vi "save_mpi_tdms.vi"(3 "System Information cluster":T1, 5 "Subject metadata cluster":T2, 7 "Device Name":tag="DAQ2", 8 "TxRxParams":T3={"sample rate"=1000000.0, "Transmit frequency"=25000.0, "Transmit amplitude"=1.577, "sample rate digital out"=40000.0, "TX cycles"=600, "sample rate DAQ1"=1000000.0, "Receive frequency"=75000.0, "Receive range"=1.0, "TX harmonics"=[50000.0, 75000.0, 100000.0, 125000.0, 150000.0, 175000.0, 200000.0, 225000.0]} {"TX harmonics" format="%#_6p"; "Receive frequency" format="%#_6p"; "sample rate DAQ1" format="%#_6p"; "sample rate digital out" format="%#_6p"; "Transmit frequency" format="%#_6p"; "sample rate" format="%#_6p"}, 9 "image dataset":string, 10 "Path":path, 11 "Cluster in":T4={"Magnitude meas."=[], "Phase meas."=[], "Shift meas."=[], "cw"=TRUE, "projections per image"=0, "ramp-up readouts"=0, "current sense type"="", "Number of pulses per image"=0, "Rotation enabled"=TRUE, "Rotary position"=[], "Baseline magnitude"=0.0, "Baseline phase"=0.0, "Wait readouts"=0, "Shift waveform type"="", "Shift enabled"=TRUE, "Time domain data"=[], "Motor pulse duration"=0.0, "Shift Amp pk"=0.0, "Shift DC offset"=0.0, "Notes"="", "Reconstructed image"=bytes[0], "Rotary encoder type"="", "Image start"=timestamp(0 s since 1904-01-01), "Image stop"=timestamp(0 s since 1904-01-01), "readouts per projection"=0, "Recon enabled"=FALSE, "Bidirectional shift"=FALSE, "Imager mode"="", "Shift delay"=0.0, "Shift frequency"=0.0, "Image time (calc)"=0.0, "Initial encoder position"=0.0, "Recon data"=[], "Trigger line values"=[], "Bed position"=0.0, "Sample image"=bytes[0], "Patch amplitude"=0.0, "Patch frequency"=0.0, "Patch phase"=0.0, "proj mag f2-f9"=[], "proj phase f2-f9"=[], "Tx waveform"=[], "Tx FFT mag"=[], "Tx FFT phase"=[], "Temps"=[]}) -> ()   [LabVIEW 2021]
uses:
  <resource>/objmgr/daqmx.rc
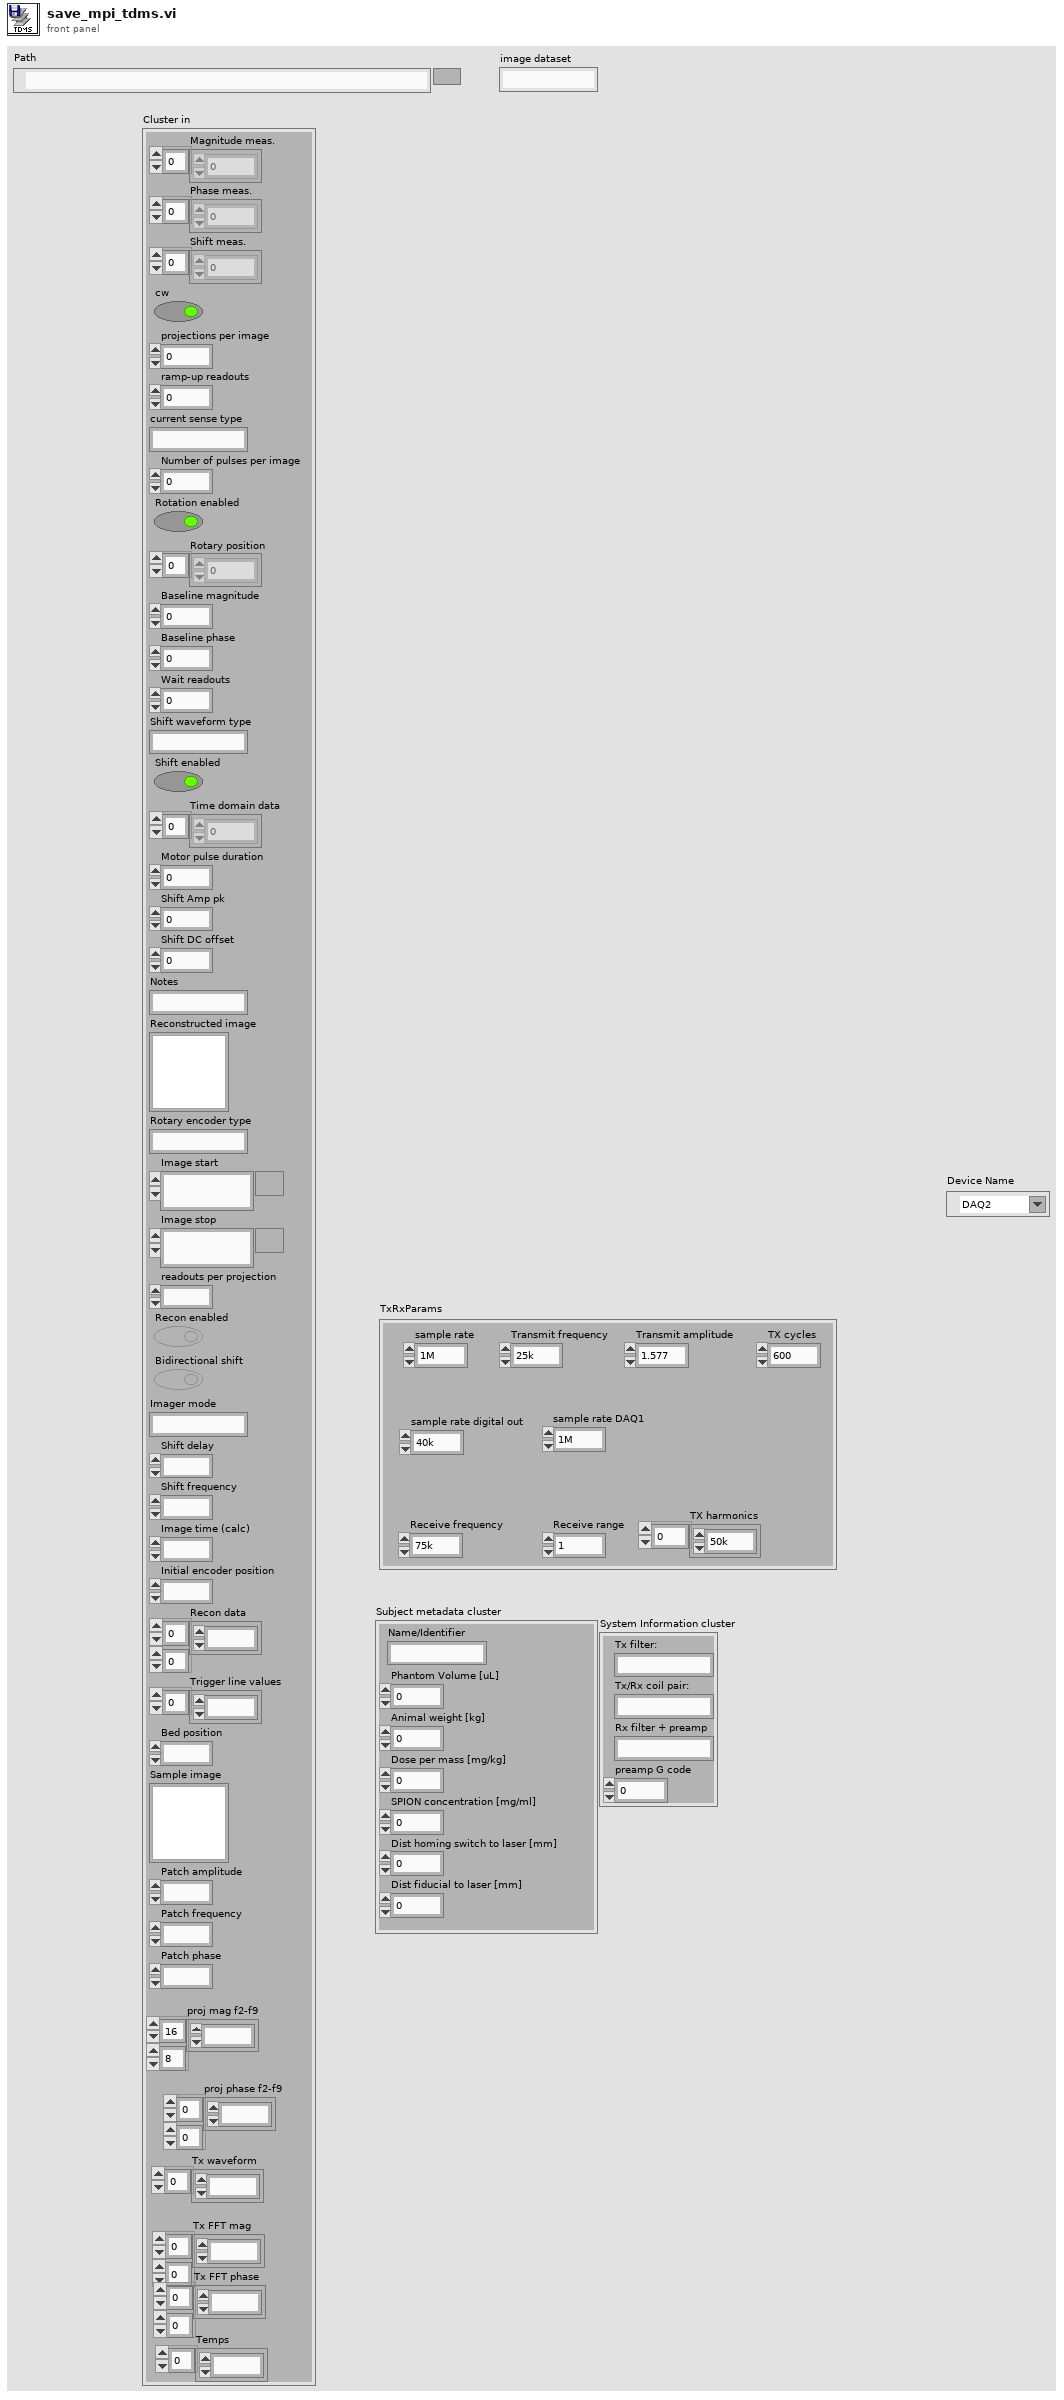
[diagram p1: front panel]
types:
  T1 = cluster{"Tx filter:":string, "Tx/Rx coil pair:":string, "Rx filter + preamp":string, "preamp G code":dbl}
  T2 = cluster{"Name/Identifier":string, "Phantom Volume [uL]":dbl, "Animal weight [kg]":dbl, "Dose per mass [mg/kg]":dbl, "SPION concentration [mg/ml]":dbl, "Dist homing switch to laser [mm]":dbl, "Dist fiducial to laser [mm]":dbl}
  T3 = cluster{"sample rate":dbl, "Transmit frequency":dbl, "Transmit amplitude":dbl, "sample rate digital out":dbl, "TX cycles":i32, "sample rate DAQ1":dbl, "Receive frequency":dbl, "Receive range":dbl, "TX harmonics":dbl[]}
  T4 = cluster{"Magnitude meas.":dbl[], "Phase meas.":dbl[], "Shift meas.":dbl[], "cw":bool, "projections per image":i32, "ramp-up readouts":i32, "current sense type":string, "Number of pulses per image":i32, "Rotation enabled":bool, "Rotary position":dbl[], "Baseline magnitude":dbl, "Baseline phase":dbl, "Wait readouts":i32, "Shift waveform type":string, "Shift enabled":bool, "Time domain data":dbl[], "Motor pulse duration":dbl, "Shift Amp pk":dbl, "Shift DC offset":dbl, "Notes":string, "Reconstructed image":picture, "Rotary encoder type":string, "Image start":timestamp, "Image stop":timestamp, "readouts per projection":i32, "Recon enabled":bool, "Bidirectional shift":bool, "Imager mode":string, "Shift delay":dbl, "Shift frequency":dbl, "Image time (calc)":dbl, "Initial encoder position":dbl, "Recon data":dbl[][], "Trigger line values":i32[], "Bed position":dbl, "Sample image":picture, "Patch amplitude":dbl, "Patch frequency":dbl, "Patch phase":dbl, "proj mag f2-f9":dbl[][], "proj phase f2-f9":dbl[][], "Tx waveform":dbl[], "Tx FFT mag":dbl[][], "Tx FFT phase":dbl[][], "Temps":dbl[]}
  T5 = enum16{"open", "open or create", "create or replace", "create", "open (read-only)"}
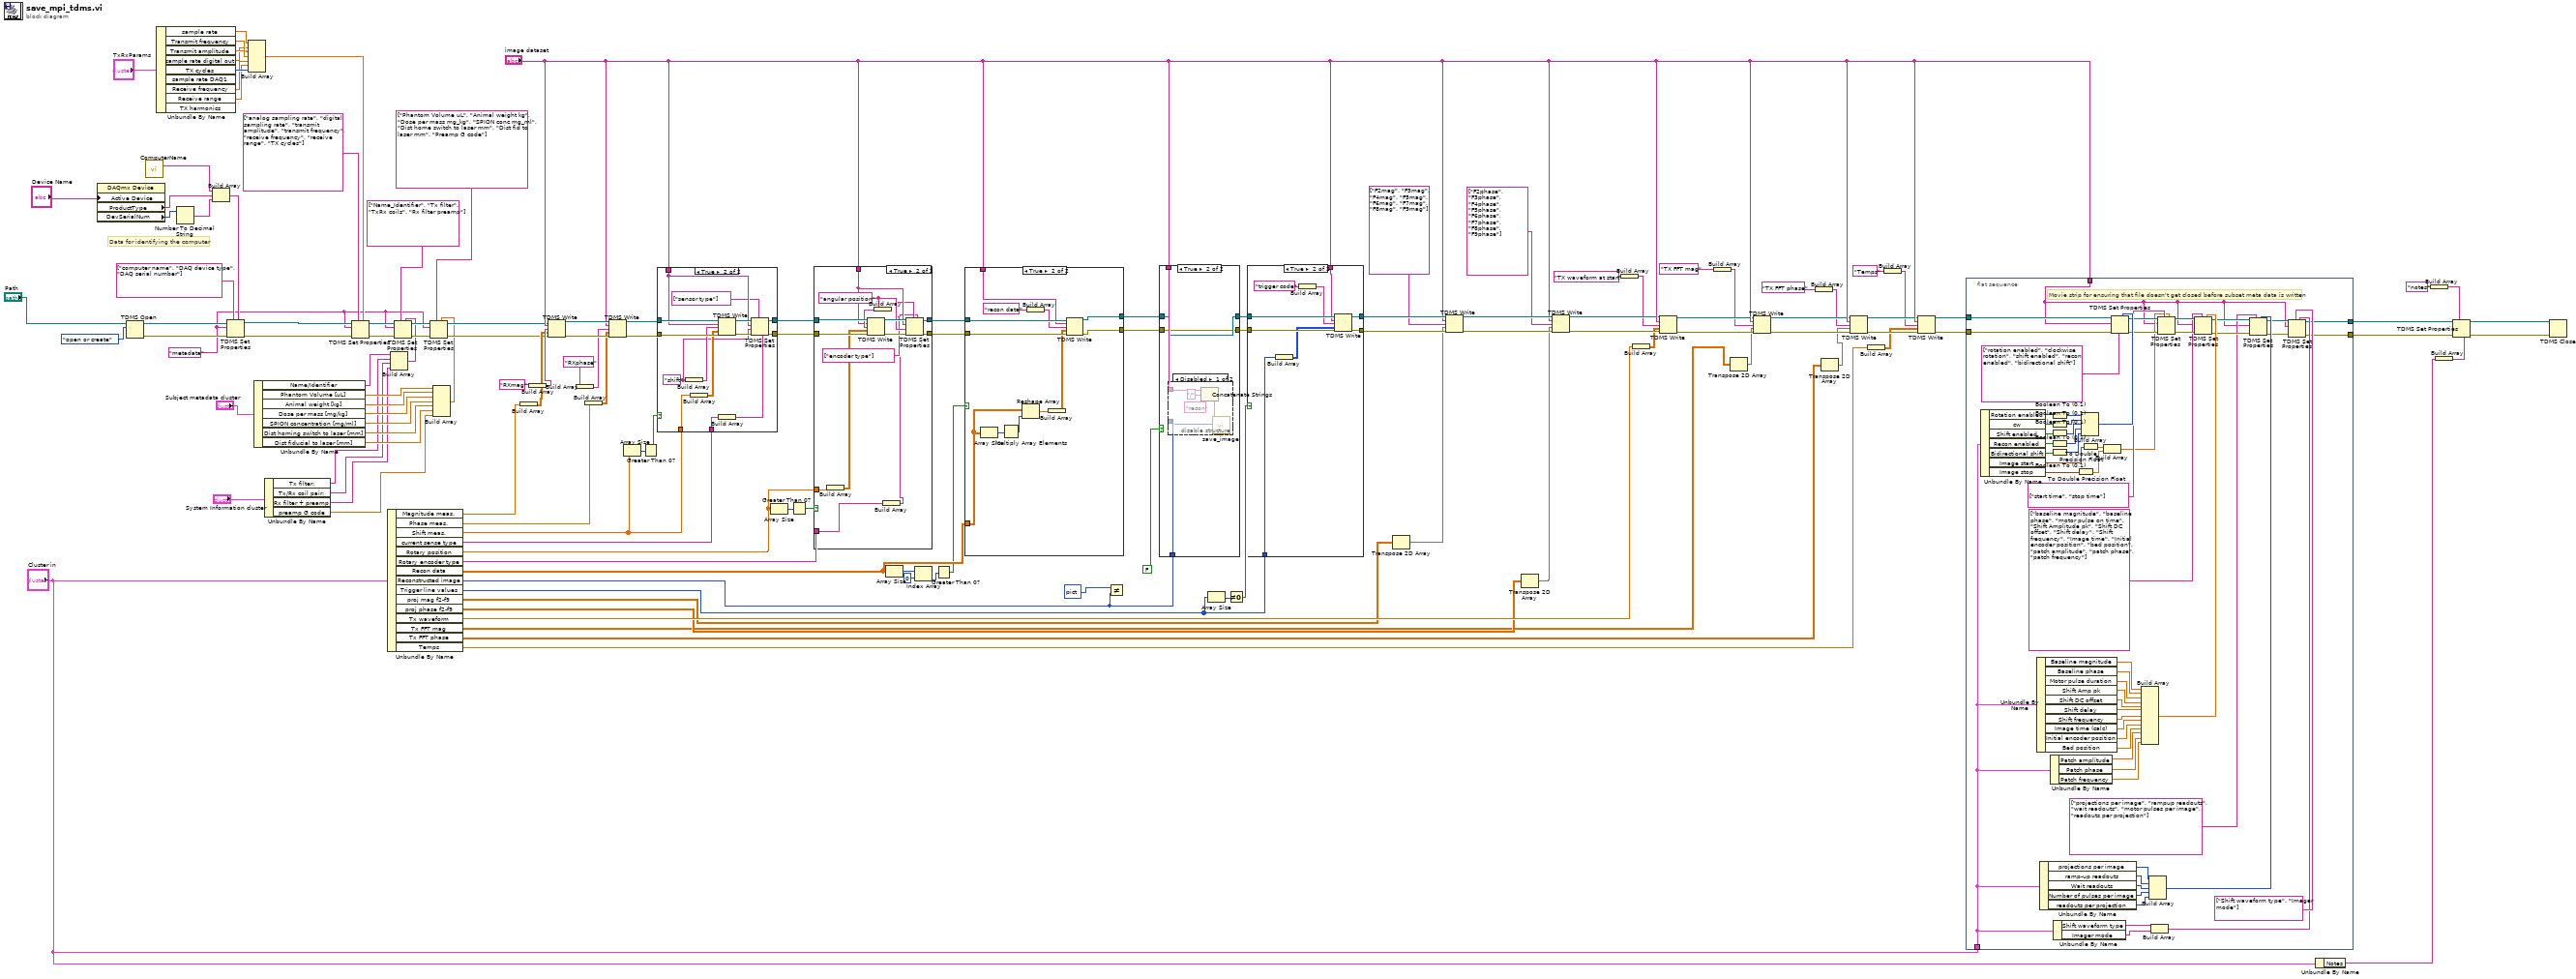
[diagram p0: block diagram]
diagram:
  w5 = "metadata" ("group name")
  # "Data for identifying the computer"
  n1 = property class="DAQmx Device"("Active Device"="Device Name") -> ("ProductType"=w130:string, "DevSerialNum"=w132:u32)  [unwired: 2 in, 2 out]
  n2 = TDMS Open(10:T5."open or create" ("operation (0:open)"), 11:"Path") -> (0:w118:errorcluster, 3:w119:refnum<k34>)  [unwired: 5 in]
  n3 = call "ComputerName.vi"() -> ("String/Binary data"=w129:string)  [unwired: 4 in, 1 out]
  n4 = Unbundle By Name("TxRxParams") -> ("sample rate"=w29:dbl, "Transmit frequency"=w32:dbl, "Transmit amplitude"=w31:dbl, "sample rate digital out"=w30:dbl, "TX cycles"=w35:i32, "Receive frequency"=w33:dbl, "Receive range"=w34:dbl)  [unwired: 2 out]
  n5 = Number To Decimal String(number=w132) -> (decimal integer string=w131:string)  [unwired: 1 in]
  n6 = Build Array(w129, w130, w131) -> (w116:string[])
  n7 = TDMS Set Properties(5:w116, 7:string[] ["computer name", "DAQ device type", "DAQ serial number"] ("Name(s)"), 8:w118, 10:w5, 11:w119) -> (0:w114:errorcluster, 3:w115:refnum<k34>)  [unwired: 1 in, 2 out]
  n8 = Build Array(w29, w30, w31, w32, w33, w34, w35) -> (w112:dbl[])
  n9 = Unbundle By Name("Subject metadata cluster") -> ("Name/Identifier"=w20:string, "Phantom Volume [uL]"=w19:dbl, "Animal weight [kg]"=w18:dbl, "Dose per mass [mg/kg]"=w17:dbl, "SPION concentration [mg/ml]"=w16:dbl, "Dist homing switch to laser [mm]"=w15:dbl, "Dist fiducial to laser [mm]"=w14:dbl)
  n10 = Unbundle By Name("System Information cluster") -> ("Tx filter:"=w9:string, "Tx/Rx coil pair:"=w8:string, "Rx filter + preamp"=w7:string, "preamp G code"=w6:dbl)
  n11 = TDMS Set Properties(5:w112, 7:string[] ["analog sampling rate", "digital sampling rate", "transmit amplitude", "transmit frequency", "receive frequency", "receive range", "TX cycles"] ("Name(s)"), 8:w114, 10:w5, 11:w115) -> (0:w27:errorcluster, 3:w28:refnum<k34>)  [unwired: 1 in, 2 out]
  n12 = Unbundle By Name("Cluster in") -> ("Magnitude meas."=w109:dbl[], "Phase meas."=w94:dbl[], "Shift meas."=w127:dbl[], "current sense type"=w90:string, "Rotary position"=w128:dbl[], "Rotary encoder type"=w89:string, "Recon data"=w122:dbl[][], "Reconstructed image"=w126:picture, "Trigger line values"=w124:i32[], "proj mag f2-f9"=w58:dbl[][], "proj phase f2-f9"=w38:dbl[][], "Tx waveform"=w72:dbl[], "Tx FFT mag"=w4:dbl[][], "Tx FFT phase"=w2:dbl[][], "Temps"=w71:dbl[])
  n13 = Build Array(w20, w9, w8, w7) -> (w22:string[])
  n14 = TDMS Set Properties(5:w22, 7:string[] ["Name_Identifier", "Tx filter", "TxRx coils", "Rx filter preamp"] ("Name(s)"), 8:w27, 10:w5, 11:w28) -> (0:w25:errorcluster, 3:w26:refnum<k34>)  [unwired: 1 in, 2 out]
  n15 = Build Array(w19, w18, w17, w16, w15, w14, w6) -> (w13:dbl[])
  n16 = TDMS Set Properties(5:w13, 7:string[] ["Phantom Volume uL", "Animal weight kg", "Dose per mass mg_kg", "SPION conc mg_ml", "Dist home switch to laser mm", "Dist fid to laser mm", "Preamp G code"] ("Name(s)"), 8:w25, 10:w5, 11:w26) -> (0:w24:errorcluster, 3:w23:refnum<k34>)  [unwired: 1 in, 2 out]
  n17 = Build Array(w109) -> (w108:dbl[][])
  n18 = Build Array("RXmag" ("string")) -> (w110:string[])
  n19 = TDMS Write(0:w23, 5:"image dataset", 7:w110, 9:w108, 11:w24) -> (4:w96:refnum<k34>, 15:w97:errorcluster)  [unwired: 1 in, 2 out]
  n20 = Build Array("RXphase" ("string")) -> (w95:string[])
  n21 = Build Array(w94) -> (w93:dbl[][])
  n22 = TDMS Write(0:w96, 5:"image dataset", 7:w95, 9:w93, 11:w97) -> (4:w92:refnum<k34>, 15:w91:errorcluster)  [unwired: 1 in, 2 out]
  n23 = Array Size(array=w127) -> (size(s)=w104:i32)
  n24 = Greater Than 0?(x=w104) -> (x > 0?=w105:bool)
  n25 = case shown="True" w105 {
    tunnel: w127 -> [_ w145]
    tunnel: "image dataset" -> [_ w141]
    tunnel: w92 -> [w134 w148]
    tunnel: w91 -> [w133 w147]
    tunnel: w90 -> [_ w138]
    tunnel: [w134 w136] -> w88
    tunnel: [w133 w135] -> w87
    frame False {
    }
    frame True {
      w140 = "shift" ("string")
      n26 = Build Array(w140) -> (w146:string[])
      n27 = Build Array(w145) -> (w144:dbl[][])
      n28 = TDMS Write(0:w148, 5:w141, 7:w146, 9:w144, 11:w147) -> (4:w143:refnum<k34>, 15:w142:errorcluster)  [unwired: 1 in, 2 out]
      n29 = Build Array(w138) -> (w137:string[])
      n30 = TDMS Set Properties(5:w137, 7:string[] ["sensor type"] ("Attribute Name(s)"), 8:w142, 9:w140, 10:w141, 11:w143) -> (0:w135:errorcluster, 3:w136:refnum<k34>)  [unwired: 2 out]
    }
  }
  n31 = Array Size(array=w128) -> (size(s)=w107:i32)
  n32 = Greater Than 0?(x=w107) -> (x > 0?=w106:bool)
  n33 = case shown="True" w106 {
    tunnel: w128 -> [_ w156]
    tunnel: "image dataset" -> [_ w154]
    tunnel: w89 -> [_ w164]
    tunnel: w88 -> [w150 w163]
    tunnel: w87 -> [w149 w162]
    tunnel: [w150 w159] -> w86
    tunnel: [w149 w158] -> w85
    frame False {
    }
    frame True {
      w153 = "angular position" ("string")
      n34 = Build Array(w156) -> (w155:dbl[][])
      n35 = Build Array(w153) -> (w157:string[])
      n36 = TDMS Write(0:w163, 5:w154, 7:w157, 9:w155, 11:w162) -> (4:w161:refnum<k34>, 15:w160:errorcluster)  [unwired: 1 in, 2 out]
      n37 = Build Array(w164) -> (w151:string[])
      n38 = TDMS Set Properties(5:w151, 7:string[] ["encoder type"] ("Attribute Name(s)"), 8:w160, 9:w153, 10:w154, 11:w161) -> (0:w158:errorcluster, 3:w159:refnum<k34>)  [unwired: 2 out]
    }
  }
  n39 = Array Size(array=w122) -> (size(s)=w102:i32[])
  n40 = Index Array(array=w102, index=0) -> (element=w100:i32)
  n41 = Greater Than 0?(x=w100) -> (x > 0?=w99:bool)
  n42 = case shown="True" w99 {
    tunnel: "image dataset" -> [_ w176]
    tunnel: w122 -> [_ w172]
    tunnel: w86 -> [w166 w178]
    tunnel: w85 -> [w165 w177]
    tunnel: [w166 w168] -> w79
    tunnel: [w165 w167] -> w78
    frame False {
    }
    frame True {
      n43 = Array Size(array=w172) -> (size(s)=w170:i32[])
      n44 = Multiply Array Elements(1:w170) -> (0:w171:i32)
      n45 = Reshape Array(w172, w171) -> (w174:dbl[])
      n46 = Build Array("recon data" ("string")) -> (w169:string[])
      n47 = Build Array(w174) -> (w173:dbl[][])
      n48 = TDMS Write(0:w178, 5:w176, 7:w169, 9:w173, 11:w177) -> (4:w168:refnum<k34>, 15:w167:errorcluster)  [unwired: 1 in, 2 out]
    }
  }
  n49 = Not Equal?(x=picture data[5B] ("Reconstructed image"), y=w126) -> ()  [unwired: 1 out]
  n50 = case shown="True" FALSE {
    tunnel: [w180 w182] -> w84
    tunnel: [w179 w181] -> w83
    tunnel: w126 -> [_ w184]
    tunnel: "image dataset" -> [_ w183]
    tunnel: w79 -> [w180 w182]
    tunnel: w78 -> [w179 w181]
    frame False {
    }
    frame True {
      n51 = disable-structure shown="Disabled" {
        disable-tunnel: w184 -> [w189 _]
        disable-tunnel: w183 -> [w186 _]
        frame Disabled {
          n52 = Concatenate Strings(w186, "/" ("string"), "recon" ("string")) -> (w185:string)
          n53 = call "save_image.vi"(9:w185, "picture"=w189) -> ()  [unwired: 10 in]
        }
        frame Enabled {
        }
      }
    }
  }
  n54 = Array Size(array=w124) -> (size(s)=w82:i32)
  n55 = Not Equal To 0?(x=w82) -> (x != 0?=w81:bool)
  n56 = case shown="True" w81 {
    tunnel: w84 -> [w191 w200]
    tunnel: w83 -> [w190 w199]
    tunnel: [w191 w198] -> w77
    tunnel: [w190 w197] -> w76
    tunnel: "image dataset" -> [_ w196]
    tunnel: w124 -> [_ w193]
    frame False {
    }
    frame True {
      n57 = Build Array(w193) -> (w192:i32[][])
      n58 = Build Array("trigger code" ("string")) -> (w194:string[])
      n59 = TDMS Write(0:w200, 5:w196, 7:w194, 9:w192, 11:w199) -> (4:w198:refnum<k34>, 15:w197:errorcluster)  [unwired: 1 in, 2 out]
    }
  }
  n60 = Transpose 2D Array(2D array=w58) -> (transposed array=w59:dbl[][])
  n61 = TDMS Write(0:w77, 5:"image dataset", 7:string[] ["F2mag", "F3mag", "F4mag", "F5mag", "F6mag", "F7mag", "F8mag", "F9mag"], 9:w59, 11:w76) -> (4:w73:refnum<k34>, 15:w74:errorcluster)  [unwired: 1 in, 2 out]
  n62 = Transpose 2D Array(2D array=w38) -> (transposed array=w37:dbl[][])
  n63 = TDMS Write(0:w73, 5:"image dataset", 7:string[] ["F2phase", "F3phase", "F4phase", "F5phase", "F6phase", "F7phase", "F8phase", "F9phase"], 9:w37, 11:w74) -> (4:w56:refnum<k34>, 15:w55:errorcluster)  [unwired: 1 in, 2 out]
  n64 = Build Array("TX waveform at start" ("string")) -> (w53:string[])
  n65 = Build Array(w72) -> (w52:dbl[][])
  n66 = TDMS Write(0:w56, 5:"image dataset", 7:w53, 9:w52, 11:w55) -> (4:w51:refnum<k34>, 15:w50:errorcluster)  [unwired: 1 in, 2 out]
  n67 = Build Array("TX FFT mag" ("string")) -> (w48:string[])
  n68 = Transpose 2D Array(2D array=w4) -> (transposed array=w3:dbl[][])
  n69 = TDMS Write(0:w51, 5:"image dataset", 7:w48, 9:w3, 11:w50) -> (4:w47:refnum<k34>, 15:w46:errorcluster)  [unwired: 1 in, 2 out]
  n70 = Build Array("TX FFT phase" ("string")) -> (w45:string[])
  n71 = Transpose 2D Array(2D array=w2) -> (transposed array=w1:dbl[][])
  n72 = TDMS Write(0:w47, 5:"image dataset", 7:w45, 9:w1, 11:w46) -> (4:w43:refnum<k34>, 15:w42:errorcluster)  [unwired: 1 in, 2 out]
  n73 = Build Array(w71) -> (w39:dbl[][])
  n74 = Build Array("Temps" ("string")) -> (w40:string[])
  n75 = TDMS Write(0:w43, 5:"image dataset", 7:w40, 9:w39, 11:w42) -> (4:w69:refnum<k34>, 15:w68:errorcluster)  [unwired: 1 in, 2 out]
  n76 = flat-sequence {
    tunnel: "Cluster in" -> [w228]
    tunnel: "image dataset" -> [w205]
    tunnel: w69 -> [w223]
    tunnel: w68 -> [w222]
    tunnel: [w202] -> w67
    tunnel: [w201] -> w66
    frame #0 {
      # "Movie strip for ensuring that file doesn't get closed before subset meta data is written"
      n77 = Unbundle By Name(w228) -> ("Rotation enabled"=w238:bool, "cw"=w235:bool, "Shift enabled"=w234:bool, "Recon enabled"=w232:bool, "Bidirectional shift"=w230:bool, "Image start"=w253:timestamp, "Image stop"=w250:timestamp)
      n78 = Unbundle By Name(w228) -> ("Baseline magnitude"=w258:dbl, "Baseline phase"=w257:dbl, "Motor pulse duration"=w256:dbl, "Shift Amp pk"=w255:dbl, "Shift DC offset"=w254:dbl, "Shift delay"=w243:dbl, "Shift frequency"=w242:dbl, "Image time (calc)"=w241:dbl, "Initial encoder position"=w239:dbl, "Bed position"=w224:dbl)
      n79 = Unbundle By Name(w228) -> ("projections per image"=w249:i32, "ramp-up readouts"=w248:i32, "Wait readouts"=w247:i32, "Number of pulses per image"=w246:i32, "readouts per projection"=w244:i32)
      n80 = Unbundle By Name(w228) -> ("Patch amplitude"=w225:dbl, "Patch phase"=w226:dbl, "Patch frequency"=w227:dbl)
      n81 = Boolean To (0,1)(Boolean=w238) -> (0, 1=w237:i16)
      n82 = Boolean To (0,1)(Boolean=w235) -> (0, 1=w236:i16)
      n83 = Boolean To (0,1)(Boolean=w234) -> (0, 1=w233:i16)
      n84 = Boolean To (0,1)(Boolean=w232) -> (0, 1=w231:i16)
      n85 = Boolean To (0,1)(Boolean=w230) -> (0, 1=w229:i16)
      n86 = Unbundle By Name(w228) -> ("Shift waveform type"=w245:string, "Imager mode"=w240:string)
      n87 = To Double Precision Float(number=w250) -> (double precision float=w251:dbl)
      n88 = Build Array(w237, w236, w233, w231, w229) -> (w220:i16[])
      n89 = To Double Precision Float(number=w253) -> (double precision float=w252:dbl)
      n90 = Build Array(w252, w251) -> (w216:dbl[])
      n91 = TDMS Set Properties(5:w220, 7:string[] ["rotation enabled", "clockwise rotation", "shift enabled", "recon enabled", "bidirectional shift"] ("Name(s)"), 8:w222, 10:w205, 11:w223) -> (0:w218:errorcluster, 3:w219:refnum<k34>)  [unwired: 1 in, 2 out]
      n92 = Build Array(w258, w257, w256, w255, w254, w243, w242, w241, w239, w224, w225, w226, w227) -> (w212:dbl[])
      n93 = Build Array(w249, w248, w247, w246, w244) -> (w208:i32[])
      n94 = Build Array(w245, w240) -> (w203:string[])
      n95 = TDMS Set Properties(5:w216, 7:string[] ["start time", "stop time"] ("Name(s)"), 8:w218, 10:w205, 11:w219) -> (0:w215:errorcluster, 3:w214:refnum<k34>)  [unwired: 1 in, 2 out]
      n96 = TDMS Set Properties(5:w212, 7:string[] ["baseline magnitude", "baseline phase", "motor pulse on time", "Shift Amplitude pk", "Shift DC offset", "Shift delay", "Shift frequency", "Image time", "Initial encoder position", "bed position", "patch amplitude", "patch phase", "patch frequency"] ("Name(s)"), 8:w215, 10:w205, 11:w214) -> (0:w210:errorcluster, 3:w211:refnum<k34>)  [unwired: 1 in, 2 out]
      n97 = TDMS Set Properties(5:w208, 7:string[] ["projections per image", "rampup readouts", "wait readouts", "motor pulses per image", "readouts per projection"] ("Name(s)"), 8:w210, 10:w205, 11:w211) -> (0:w206:errorcluster, 3:w207:refnum<k34>)  [unwired: 1 in, 2 out]
      n98 = TDMS Set Properties(5:w203, 7:string[] ["Shift waveform type", "Imager mode"] ("Name(s)"), 8:w206, 10:w205, 11:w207) -> (0:w201:errorcluster, 3:w202:refnum<k34>)  [unwired: 1 in, 2 out]
    }
  }
  n99 = Unbundle By Name("Cluster in") -> ("Notes"=w62:string)
  n100 = Build Array("notes" ("Dataset Path")) -> (w65:string[])
  n101 = Build Array(w62) -> (w63:string[])
  n102 = TDMS Set Properties(5:w63, 7:w65, 8:w66, 11:w67) -> (0:w60:errorcluster, 3:w61:refnum<k34>)  [unwired: 2 in, 2 out]
  n103 = TDMS Close(8:w60, 11:w61) -> ()  [unwired: 2 out]
